vi "Dummy Dialog.vi"   [LabVIEW 2014]
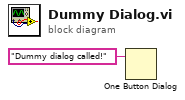
[diagram p0: block diagram]
diagram:
  n1 = One Button Dialog(message="Dummy dialog called!") -> ()  [unwired: 1 in, 1 out]
